vi "Save zero position.vi"(8 "error in (no error)":errorcluster, 11 "Zero position":cluster{"M1":dbl, "M2":dbl}) -> (0 "error out":errorcluster)   [LabVIEW 2020]
uses:
  <vilib>/Utility/config.llb/NI_LVConfig.lvlib
  <vilib>/Utility/config.llb/Write Key (Double).vi
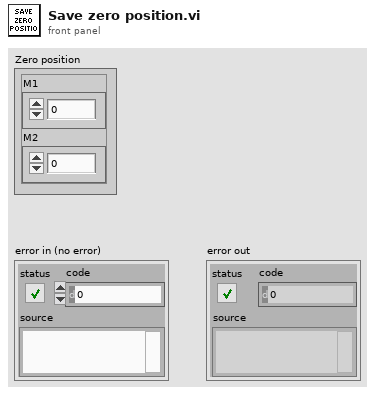
[diagram p1: front panel]
types:
  T1 = typedef "NI_LVConfig.lvlib/Config Data RefNum.ctl" = refnum<k1>
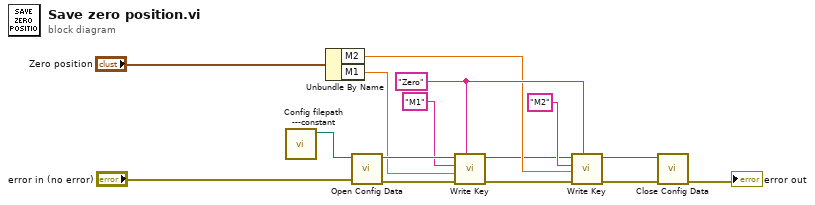
[diagram p0: block diagram]
diagram:
  w7 = "Zero" ("section")
  n1 = call "Config filepath ---constant.vi"() -> ("config file path"=w1:path)  [unwired: 11 in]
  n2 = Unbundle By Name("Zero position") -> ("M2"=w5:dbl, "M1"=w10:dbl)
  n3 = call <vilib>:"Open Config Data.vi"("error in (no error)"="error in (no error)", "configuration file path"=w1) -> ("error out"=w14:errorcluster, "refnum"=w13:T1)  [unwired: 7 in, 1 out]
  n4 = call-poly <vilib>:"Write Key.vi"("section"=w7, "error in (no error)"=w14, "value"=w10, "key"="M1", "refnum"=w13) -> ("error out"=w9:errorcluster, "refnum out"=w2:T1)  [unwired: 4 in, 1 out]
  n5 = call-poly <vilib>:"Write Key.vi"("section"=w7, "error in (no error)"=w9, "value"=w5, "key"="M2", "refnum"=w2) -> ("error out"=w8:errorcluster, "refnum out"=w3:T1)  [unwired: 4 in, 1 out]
  n6 = call <vilib>:"Close Config Data.vi"("error in (no error)"=w8, "refnum"=w3) -> ("error out"=→"error out":errorcluster)  [unwired: 8 in, 1 out]
